vi "add tag to table.vi"(8 "error in":errorcluster, 10 "system tag":refnum<class "data bus tag description.lvclass">, 11 "data table in":T1) -> (0 "error out":errorcluster, 2 "new index":i32, 3 "data table out":T1)   [LabVIEW 2013, in "data bus values.lvlib"]
doc: "Adds a tag to a data table."
uses:
  data bus values.lvlib
  data table.ctl
  tag/data bus tag description.lvclass
  tag/data bus tag description.lvclass/data bus tag description.ctl
  tag/read raw default value.vi
  tag/default value polymorphs/read default value Double.vi
  tag/default value polymorphs/read default value I64.vi
  tag/default value polymorphs/read default value Boolean.vi
  tag/default value polymorphs/read default value Array of Double.vi
  tag/default value polymorphs/read default value Array of I64.vi
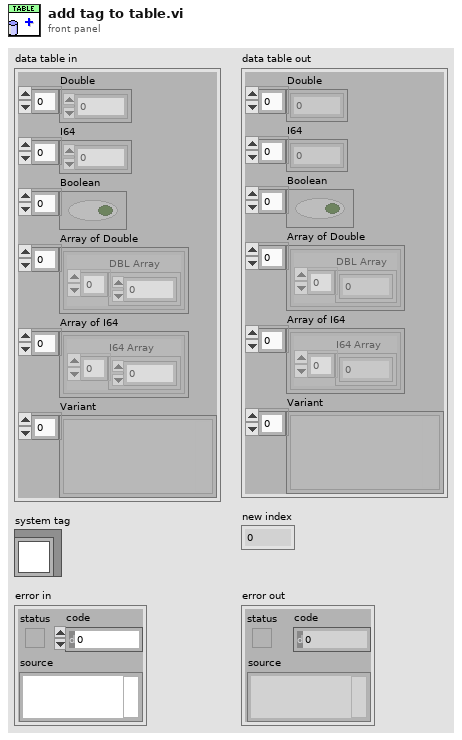
[diagram p1: front panel]
types:
  T1 = typedef "data bus values.lvlib/data table.ctl" = cluster{"Double":dbl[], "I64":i64[], "Boolean":bool[], "Array of Double":cluster{"DBL Array":dbl[]}[], "Array of I64":cluster{"I64 Array":i64[]}[], "Variant":variant[]}
  T2 = typedef "data bus tag description.lvclass/Data Type.ctl" = enum16{"Double", "I64", "Boolean", "Array of Double", "Array of I64", "Variant"}
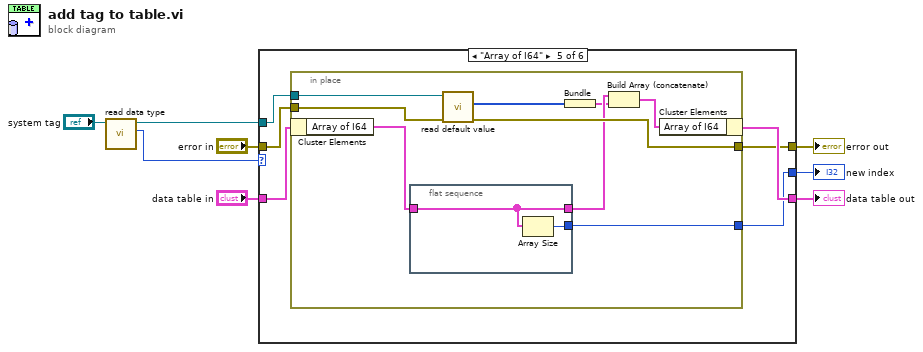
[diagram p0: block diagram]
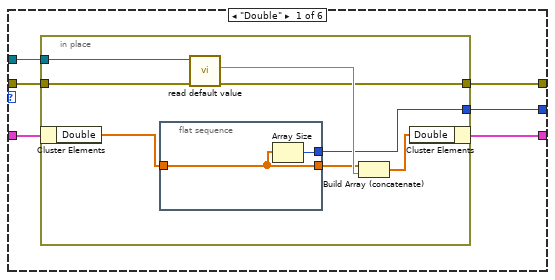
[diagram p2: hidden frame]
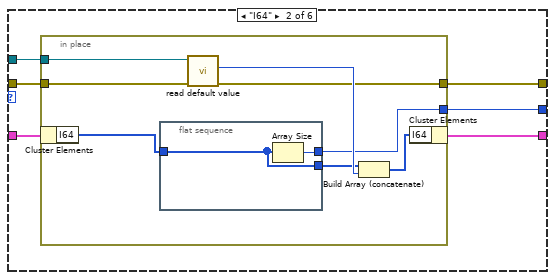
[diagram p3: hidden frame]
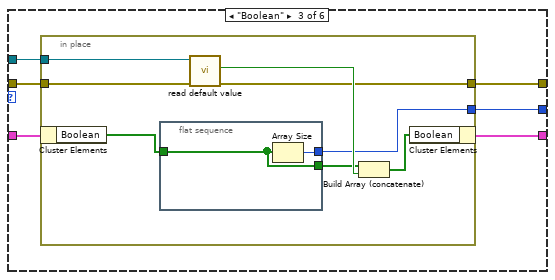
[diagram p4: hidden frame]
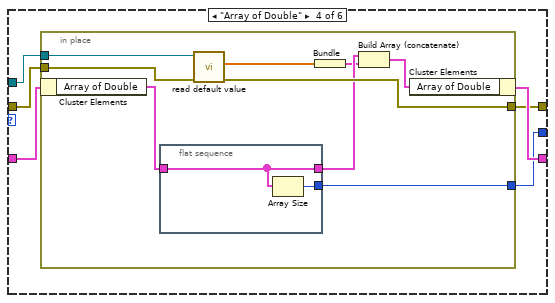
[diagram p5: hidden frame]
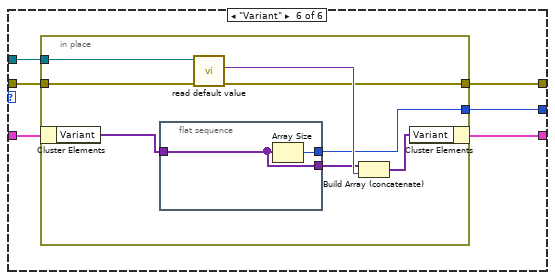
[diagram p6: hidden frame]
diagram:
  n1 = call "read data type.vi"("system tag in"="system tag") -> ("data type"=w7:T2, "system tag out"=w4:refnum<class "data bus tag description.lvclass">)  [unwired: 8 in, 1 out]
  n2 = case shown="\"Array of I64\"" w7 {
    tunnel: "data table in" -> [w14 w30 w46 w62 w79 w96]
    tunnel: [w13 w29 w45 w61 w78 w95] -> w5
    tunnel: w4 -> [w12 w28 w44 w60 w77 w94]
    tunnel: "error in" -> [w11 w27 w43 w59 w76 w93]
    tunnel: [w10 w26 w42 w58 w75 w92] -> w2
    tunnel: [w9 w25 w41 w57 w74 w91] -> w1
    frame "Double" {
      n3 = in-place {
        in-place-border: w12 -> [w22]
        in-place-border: w11 -> [w20]
        in-place-border: [w18] -> w10
        in-place-border: [w15] -> w9
        n4 = in-place-cluster #1(w14) -> ("Double"=w17:dbl[])
        n5 = flat-sequence {
          tunnel: w17 -> [w24]
          tunnel: [w24] -> w16
          tunnel: [w23] -> w15
          frame #0 {
            n6 = Array Size(array=w24) -> (size(s)=w23:i32)
          }
        }
        n7 = call-poly "read default value.vi"("error in"=w20, "system tag in"=w22) -> ("error out"=w18:errorcluster, "default value"=w21:dbl)  [unwired: 6 in, 2 out]
        n8 = Build Array (concatenate)(w16, w21) -> (w19:dbl[])
        n9 = in-place-cluster #1("Double"=w19) -> (w13:T1)
      }
    }
    frame "I64" {
      n10 = in-place {
        in-place-border: w28 -> [w38]
        in-place-border: w27 -> [w36]
        in-place-border: [w34] -> w26
        in-place-border: [w31] -> w25
        n11 = in-place-cluster #2(w30) -> ("I64"=w33:i64[])
        n12 = flat-sequence {
          tunnel: w33 -> [w40]
          tunnel: [w40] -> w32
          tunnel: [w39] -> w31
          frame #0 {
            n13 = Array Size(array=w40) -> (size(s)=w39:i32)
          }
        }
        n14 = call-poly "read default value.vi"("error in"=w36, "system tag in"=w38) -> ("error out"=w34:errorcluster, "default value"=w37:i64)  [unwired: 6 in, 2 out]
        n15 = Build Array (concatenate)(w32, w37) -> (w35:i64[])
        n16 = in-place-cluster #2("I64"=w35) -> (w29:T1)
      }
    }
    frame "Boolean" {
      n17 = in-place {
        in-place-border: w44 -> [w54]
        in-place-border: w43 -> [w52]
        in-place-border: [w50] -> w42
        in-place-border: [w47] -> w41
        n18 = in-place-cluster #3(w46) -> ("Boolean"=w49:bool[])
        n19 = flat-sequence {
          tunnel: w49 -> [w56]
          tunnel: [w56] -> w48
          tunnel: [w55] -> w47
          frame #0 {
            n20 = Array Size(array=w56) -> (size(s)=w55:i32)
          }
        }
        n21 = call-poly "read default value.vi"("error in"=w52, "system tag in"=w54) -> ("error out"=w50:errorcluster, "default value"=w53:bool)  [unwired: 6 in, 2 out]
        n22 = Build Array (concatenate)(w48, w53) -> (w51:bool[])
        n23 = in-place-cluster #3("Boolean"=w51) -> (w45:T1)
      }
    }
    frame "Array of Double" {
      n24 = in-place {
        in-place-border: w60 -> [w71]
        in-place-border: w59 -> [w69]
        in-place-border: [w67] -> w58
        in-place-border: [w64] -> w57
        n25 = in-place-cluster #4(w62) -> ("Array of Double"=w66:cluster{"DBL Array":dbl[]}[])
        n26 = flat-sequence {
          tunnel: w66 -> [w73]
          tunnel: [w73] -> w65
          tunnel: [w72] -> w64
          frame #0 {
            n27 = Array Size(array=w73) -> (size(s)=w72:i32)
          }
        }
        n28 = call-poly "read default value.vi"("error in"=w69, "system tag in"=w71) -> ("error out"=w67:errorcluster, "default value"=w70:dbl[])  [unwired: 6 in, 2 out]
        n29 = Bundle("default value"=w70) -> (w63:cluster{"default value":dbl[]})  [unwired: 1 in]
        n30 = Build Array (concatenate)(w65, w63) -> (w68:cluster{"default value":dbl[]}[])
        n31 = in-place-cluster #4("Array of Double"=w68) -> (w61:T1)
      }
    }
    frame "Array of I64" {
      n32 = in-place {
        in-place-border: w77 -> [w88]
        in-place-border: w76 -> [w86]
        in-place-border: [w84] -> w75
        in-place-border: [w81] -> w74
        n33 = in-place-cluster #5(w79) -> ("Array of I64"=w83:cluster{"I64 Array":i64[]}[])
        n34 = flat-sequence {
          tunnel: w83 -> [w90]
          tunnel: [w90] -> w82
          tunnel: [w89] -> w81
          frame #0 {
            n35 = Array Size(array=w90) -> (size(s)=w89:i32)
          }
        }
        n36 = call-poly "read default value.vi"("error in"=w86, "system tag in"=w88) -> ("error out"=w84:errorcluster, "default value"=w87:i64[])  [unwired: 6 in, 2 out]
        n37 = Bundle("default value"=w87) -> (w80:cluster{"default value":i64[]})  [unwired: 1 in]
        n38 = Build Array (concatenate)(w82, w80) -> (w85:cluster{"default value":i64[]}[])
        n39 = in-place-cluster #5("Array of I64"=w85) -> (w78:T1)
      }
    }
    frame "Variant" {
      n40 = in-place {
        in-place-border: w94 -> [w104]
        in-place-border: w93 -> [w102]
        in-place-border: [w100] -> w92
        in-place-border: [w97] -> w91
        n41 = in-place-cluster #6(w96) -> ("Variant"=w99:variant[])
        n42 = flat-sequence {
          tunnel: w99 -> [w106]
          tunnel: [w106] -> w98
          tunnel: [w105] -> w97
          frame #0 {
            n43 = Array Size(array=w106) -> (size(s)=w105:i32)
          }
        }
        n44 = call-poly "read default value.vi"("error in"=w102, "system tag in"=w104) -> ("error out"=w100:errorcluster, "raw default"=w103:variant)  [unwired: 7 in, 1 out]
        n45 = Build Array (concatenate)(w98, w103) -> (w101:variant[])
        n46 = in-place-cluster #6("Variant"=w101) -> (w95:T1)
      }
    }
  }
  "error out" <- w2
  "data table out" <- w5
  "new index" <- w1
